vi "Event Handler.vi"() -> ()   [LabVIEW 2015]
uses:
  <vilib>/Utility/miscctls.llb/LVPoint32TypeDef.ctl
panel:
  out "Coords":T1
  out "current time":timestamp
  in  "Time Check":bool
  out "Iteration":i32
  in  "Stop":bool
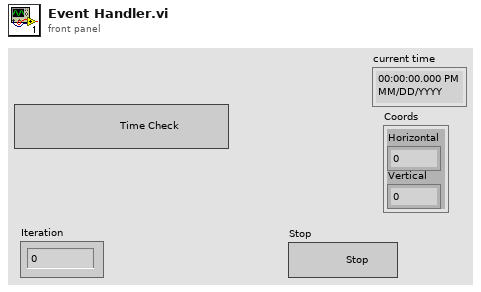
[diagram p1: front panel]
types:
  T1 = typedef "LVPoint32TypeDef.ctl" = cluster{"Horizontal":i32, "Vertical":i32}
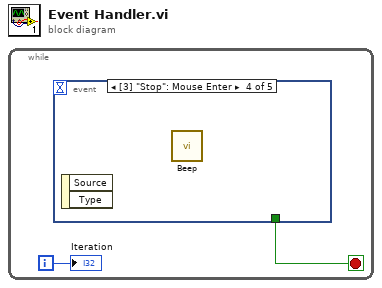
[diagram p0: block diagram]
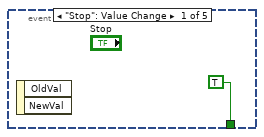
[diagram p2: hidden frame]
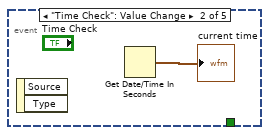
[diagram p3: hidden frame]
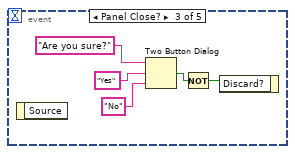
[diagram p4: hidden frame]
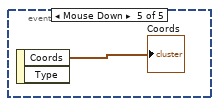
[diagram p5: hidden frame]
diagram:
  n1 = while {
    i -> [w2]
    stop <- w1 stop-if-true
    n2 = event shown="[3] \"Stop\": Mouse Enter" {
      selector: _ -> [_ _ _ _ _]
      dyn-events: _ -> [_ _ _ _ _]
      timeout: _ -> [_ _ _ _ _]
      tunnel: [TRUE _ _ _ _] -> w1
      event "Stop": Value Change {
        n3 = event-data() -> ()  [unwired: 1 in, 2 out]
      }
      event "Time Check": Value Change {
        n4 = event-data() -> ()  [unwired: 1 in, 2 out]
        n5 = Get Date/Time In Seconds() -> (seconds since 1Jan1904=→"current time":timestamp)
      }
      event Panel Close? {
        n6 = event-data() -> ()  [unwired: 1 in, 1 out]
        n7 = Two Button Dialog(message="Are you sure?", 1:"No", 2:"Yes") -> (T button?=w6:bool)
        n8 = Not(x=w6) -> (.not. x?=w5:bool)
        n9 = event-data("Discard?"=w5) -> ()  [unwired: 1 in, 1 out]
      }
      event "Stop": Mouse Enter {
        n10 = event-data() -> ()  [unwired: 1 in, 2 out]
        n11 = call <vilib>:"Beep.vi"() -> ()  [unwired: 12 in]
      }
      event Mouse Down {
        n12 = event-data() -> ("Coords"=→"Coords":T1)  [unwired: 1 in, 1 out]
      }
    }
    "Iteration" <- w2
  }
